vi "App Start.vi"(8 "error in (no error)":errorcluster, 10 "Core APIs":T1, 11 "DemoApp in":refnum<class "DemoApp.lvclass">) -> (0 "error out":errorcluster, 3 "DemoApp out":refnum<class "DemoApp.lvclass">)   [LabVIEW 2020, in "VolatusDemo.lvlib" / "DemoApp.lvclass"]
uses:
  DemoApp.lvclass
  Volatus/Core APIs.ctl
  Volatus/VolatusAPI/VolatusAPI.lvclass
  Volatus/Event API/EventAPI.lvclass
  Volatus/ConfigAPI/ConfigAPI.lvclass
  Volatus/Volatus.lvlib
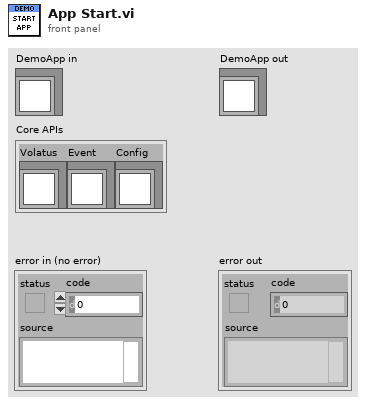
[diagram p1: front panel]
types:
  T1 = typedef "Volatus.lvlib/Core APIs.ctl" = cluster{"Volatus":refnum<class "VolatusAPI.lvclass">, "Event":refnum<class "EventAPI.lvclass">, "Config":refnum<class "ConfigAPI.lvclass">}
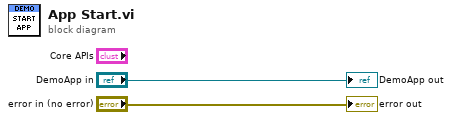
[diagram p0: block diagram]
diagram:
  "error out" <- "error in (no error)"
  "DemoApp out" <- "DemoApp in"
